vi "pp2_cam_display.vi"(0 "Image Ctl Refnum":refnum<vi>, 2 "Log File Directory":refnum<vi>, 5 "Image Memory":T2, 7 "State info Refnum":refnum<vi>, 9 "Webcam Session In":T1, 11 "error in":errorcluster) -> (15 "error out":errorcluster)   [LabVIEW 2013]
doc: "This VI is a general VI that loops through webcam images, and saves when necessary. It should be run asynchronously, so that webcam display/logging is independent of the main loop. Terminate this VI by setting the \"Webcam on\" value within the state info refnum to False."
uses:
  pp2_CTL_StateInfo.ctl
  pp2_CTL_State.ctl
  pp2_Trial.ctl
  pp2_CTL_TrialType.ctl
  labolabo2/waveforms/WFTypes.ctl
  <vilib>/vision/Image Controls.llb/IMAQ Image.ctl
  <vilib>/userdefined/High Color/IMAQdx.ctl
  <vilib>/vision/driver/NI_Vision_Acquisition_Software.lvlib
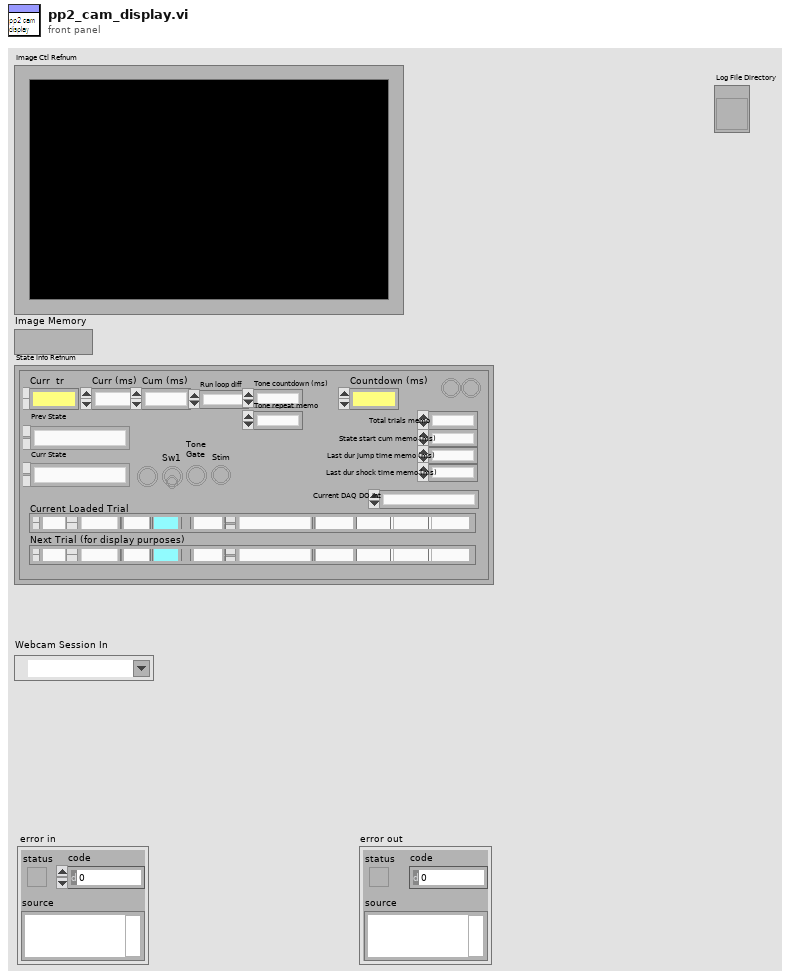
[diagram p1: front panel]
types:
  T1 = typedef "IMAQdx.ctl" = refnum<k21>
  T2 = typedef "IMAQ Image.ctl" = refnum<image>
  T3 = typedef "pp2_CTL_StateInfo.ctl" = cluster{"Curr  tr":u16, "Curr (ms)":i64, "Cum (ms)":i64, "Run loop diff":i64, "Tone countdown (ms)":i64, "Countdown (ms)":i64, "Curr State":T4, "Prev State":T4, "Null":bool, "Sw1":bool, "Sw2":bool, "Tone\nGate":bool, "Stim":bool, "Current DAQ DO Int":u16, "Current Loaded Trial":T5, "Next Trial (for display purposes)":T5, "Total trials memo":i64, "State start cum memo (ms)":i64, "Last dur jump time memo (ms)":i64, "Last dur shock time memo (ms)":i64, "Tone repeat memo":i64, "Webcam on":bool, "Webcam recording":bool}
  T4 = typedef "pp2_CTL_State.ctl" = enum8{"0 NULL", "1 Habituation", "2 (Load Trial)", "3 Stay Period", "4 (Load Audio)", "5 GO Trial", "6 GO Jumped", "7 GO Timeout", "8 NOGO Trial", "9 NOGO Jumped", "10 NOGO Timeout", "11 TEST Trial", "12 TEST Jumped", "13 TEST Timeout", "14 Intertrial Interval", "15 Done"}
  T5 = typedef "pp2_Trial.ctl" = cluster{"Trial Type Number":u8, "Trial Type":T6, "Trial Weight":u32, "Shock (mA)":dbl, "Duration (ms)":dbl, "Sound Type":T7, "Stim P1":dbl, "Stim P2":dbl, "Stim P3":dbl, "Stim P4":dbl}
  T6 = typedef "pp2_CTL_TrialType.ctl" = enum16{"OFF", "GO", "NOGO", "TEST"}
  T7 = typedef "WFTypes.ctl" = enum16{"00 NULL", "01 DC", "02 Noise", "03 Pure Tone", "04 FM Sweep"}
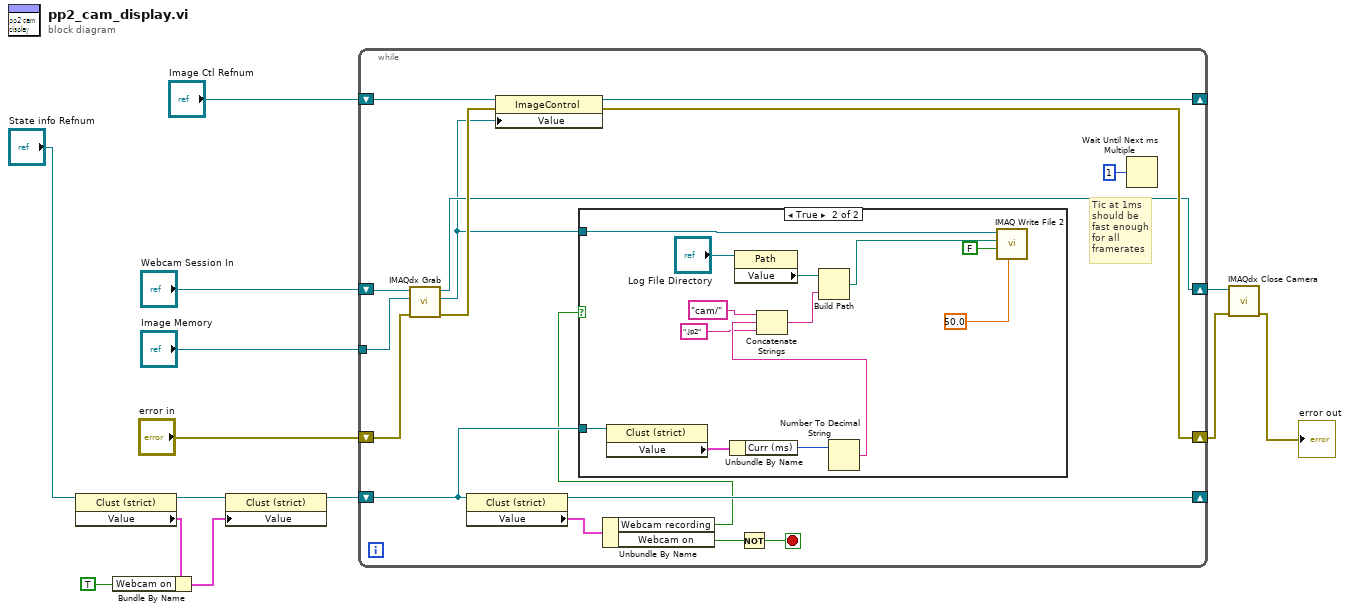
[diagram p0: block diagram]
diagram:
  n1 = property class="Clust (strict)"(reference="State info Refnum") -> (reference out=w3:refnum<vi>, "Value"=w5:T3)  [unwired: 1 in, 1 out]
  n2 = Bundle By Name(cluster=w5, "Webcam on"=TRUE) -> (w2:T3)
  n3 = property class="Clust (strict)"(reference=w3, "Value"=w2) -> (reference out=w1:refnum<vi>)  [unwired: 1 in, 1 out]
  n4 = while {
    shift-right: [w24] -> w10
    shift-left: "Webcam Session In" -> [w25]
    tunnel: "Image Memory" -> [w29]
    shift-right: [w26] -> w9
    shift-left: "error in" -> [w28]
    shift-right: [w19] -> _
    shift-left: "Image Ctl Refnum" -> [w20]
    shift-right: [w18] -> _
    shift-left: w1 -> [w15]
    stop <- w21 stop-if-true
    # "Tic at 1ms\nshould be\nfast enough\nfor all\nframerates"
    n5 = call <vilib>:"IMAQdx Grab.vi"("error in"=w28, "Image In"=w29, "Session In"=w25) -> ("error out"=w27:errorcluster, "Image Out"=w16:T2, "Session Out"=w24:T1)  [unwired: 5 in, 1 out]
    n6 = property class="Clust (strict)"(reference=w15) -> (reference out=w18:refnum<vi>, "Value"=w23:T3)  [unwired: 1 in, 1 out]
    n7 = property class="ImageControl"(reference=w20, error in=w27, "Value"=w16) -> (reference out=w19:refnum<vi>, error out=w26:errorcluster)
    n8 = Unbundle By Name(w23) -> ("Webcam recording"=w14:bool, "Webcam on"=w22:bool)
    n9 = case shown="True" w14 {
      tunnel: w16 -> [_ w31]
      tunnel: w15 -> [_ w39]
      frame False {
      }
      frame True {
        n10 = property class="Clust (strict)"(reference=w39) -> ("Value"=w38:T3)  [unwired: 1 in, 2 out]
        n11 = Unbundle By Name(w38) -> ("Curr (ms)"=w37:i64)
        n12 = property class="Path"(reference="Log File Directory") -> ("Value"=w41:path)  [unwired: 1 in, 2 out]
        n13 = Number To Decimal String(number=w37) -> (decimal integer string=w36:string)  [unwired: 1 in]
        n14 = Concatenate Strings("cam/", w36, ".jp2" ("string")) -> (w34:string)
        n15 = Build Path(base path=w41, name or relative path=w34) -> (appended path=w33:path)
        n16 = call-poly "IMAQ Write File 2"("Compression Ratio"=sgl 50.0, "Lossless? (true)"=FALSE, "File Path"=w33, "Image"=w31) -> ()  [unwired: 6 in, 2 out]
      }
    }
    n17 = Not(x=w22) -> (.not. x?=w21:bool)
    n18 = Wait Until Next ms Multiple(millisecond multiple=u32 1) -> ()  [unwired: 1 out]
  }
  n19 = call <vilib>:"IMAQdx Close Camera.vi"("error in"=w9, "Session In"=w10) -> ("error out"=→"error out":errorcluster)  [unwired: 9 in]
